vi "AA.vi"(0 "Archivo de\nreferencias (.csv)":path, 5 "ARCHIVO\nTDMS":path, 7 "Largo de ventada temporal en N samples":dbl=44100.0, 9 "Canal":string[](array[string])=["Sound Pressure_0"], 11 "frequency range":T3={"low band"=enum."20 Hz", "high band"=enum."20000 Hz"}) -> (6 "TO CSV.":string[][](array[string]))   [LabVIEW 2017]
uses:
  <vilib>/Waveform/WDTOps.llb/WDT Get Waveform Subset DBL.vi
  <vilib>/addons/Sound and Vibration/svt_Weighting/SVT A, B, C Weighting Filter (Fixed Rates) (1 Ch).vi
  <vilib>/addons/Sound and Vibration/svt_Octave_2014 standard/SVT Third-octave Analysis (1 Ch).vi
  <vilib>/addons/Sound and Vibration/svt_Octave_2014 standard/SVT Weighting Filter (octave) (1 Ch).vi
  <vilib>/addons/Sound and Vibration/svt_Level/SVT Sound Level (1 Ch).vi
  <vilib>/addons/Sound and Vibration/svt_Octave/SoundVib_Octave_2014 standard.lvlib
  <vilib>/addons/Sound and Vibration/svt_Level/SoundVib_SoundLevel.lvlib
  <vilib>/addons/Sound and Vibration/svt_Weighting/SoundVib_ABCWeighting.lvlib
panel:
  in  "reset filter (F)":bool=TRUE
  in  "dB On (T)":bool=TRUE
  in  "restart averaging\n L_bands":bool=TRUE
  in  "exp avg settings":T1={" mode"=enum."Slow", "time constant [ms]"=125.0} {"time constant [ms]" format="%.2f"}
  out "size\nSalida":i32[](array[numeric])
  out "# obs\nBands":i32[](array[numeric])
  out "# obs\nLevels A":i32
  out "total band\npower from 1/3":dbl format="%.2f"
  out "Multiplot \noctave graph 2":T2(graph)
  out "Levels_from SLM":dbl[](array[numeric])
  out "Para el CSV, excepto fecha y hora":string[][](array[string])
  out "ETIQUETAS":string[](array[string])
  out "BANDAS":dbl[][](array[numeric])
  out "Samples \npor Objeto":waveform(dbl)
  out "Secciones":waveform(dbl)[](array[waveform])
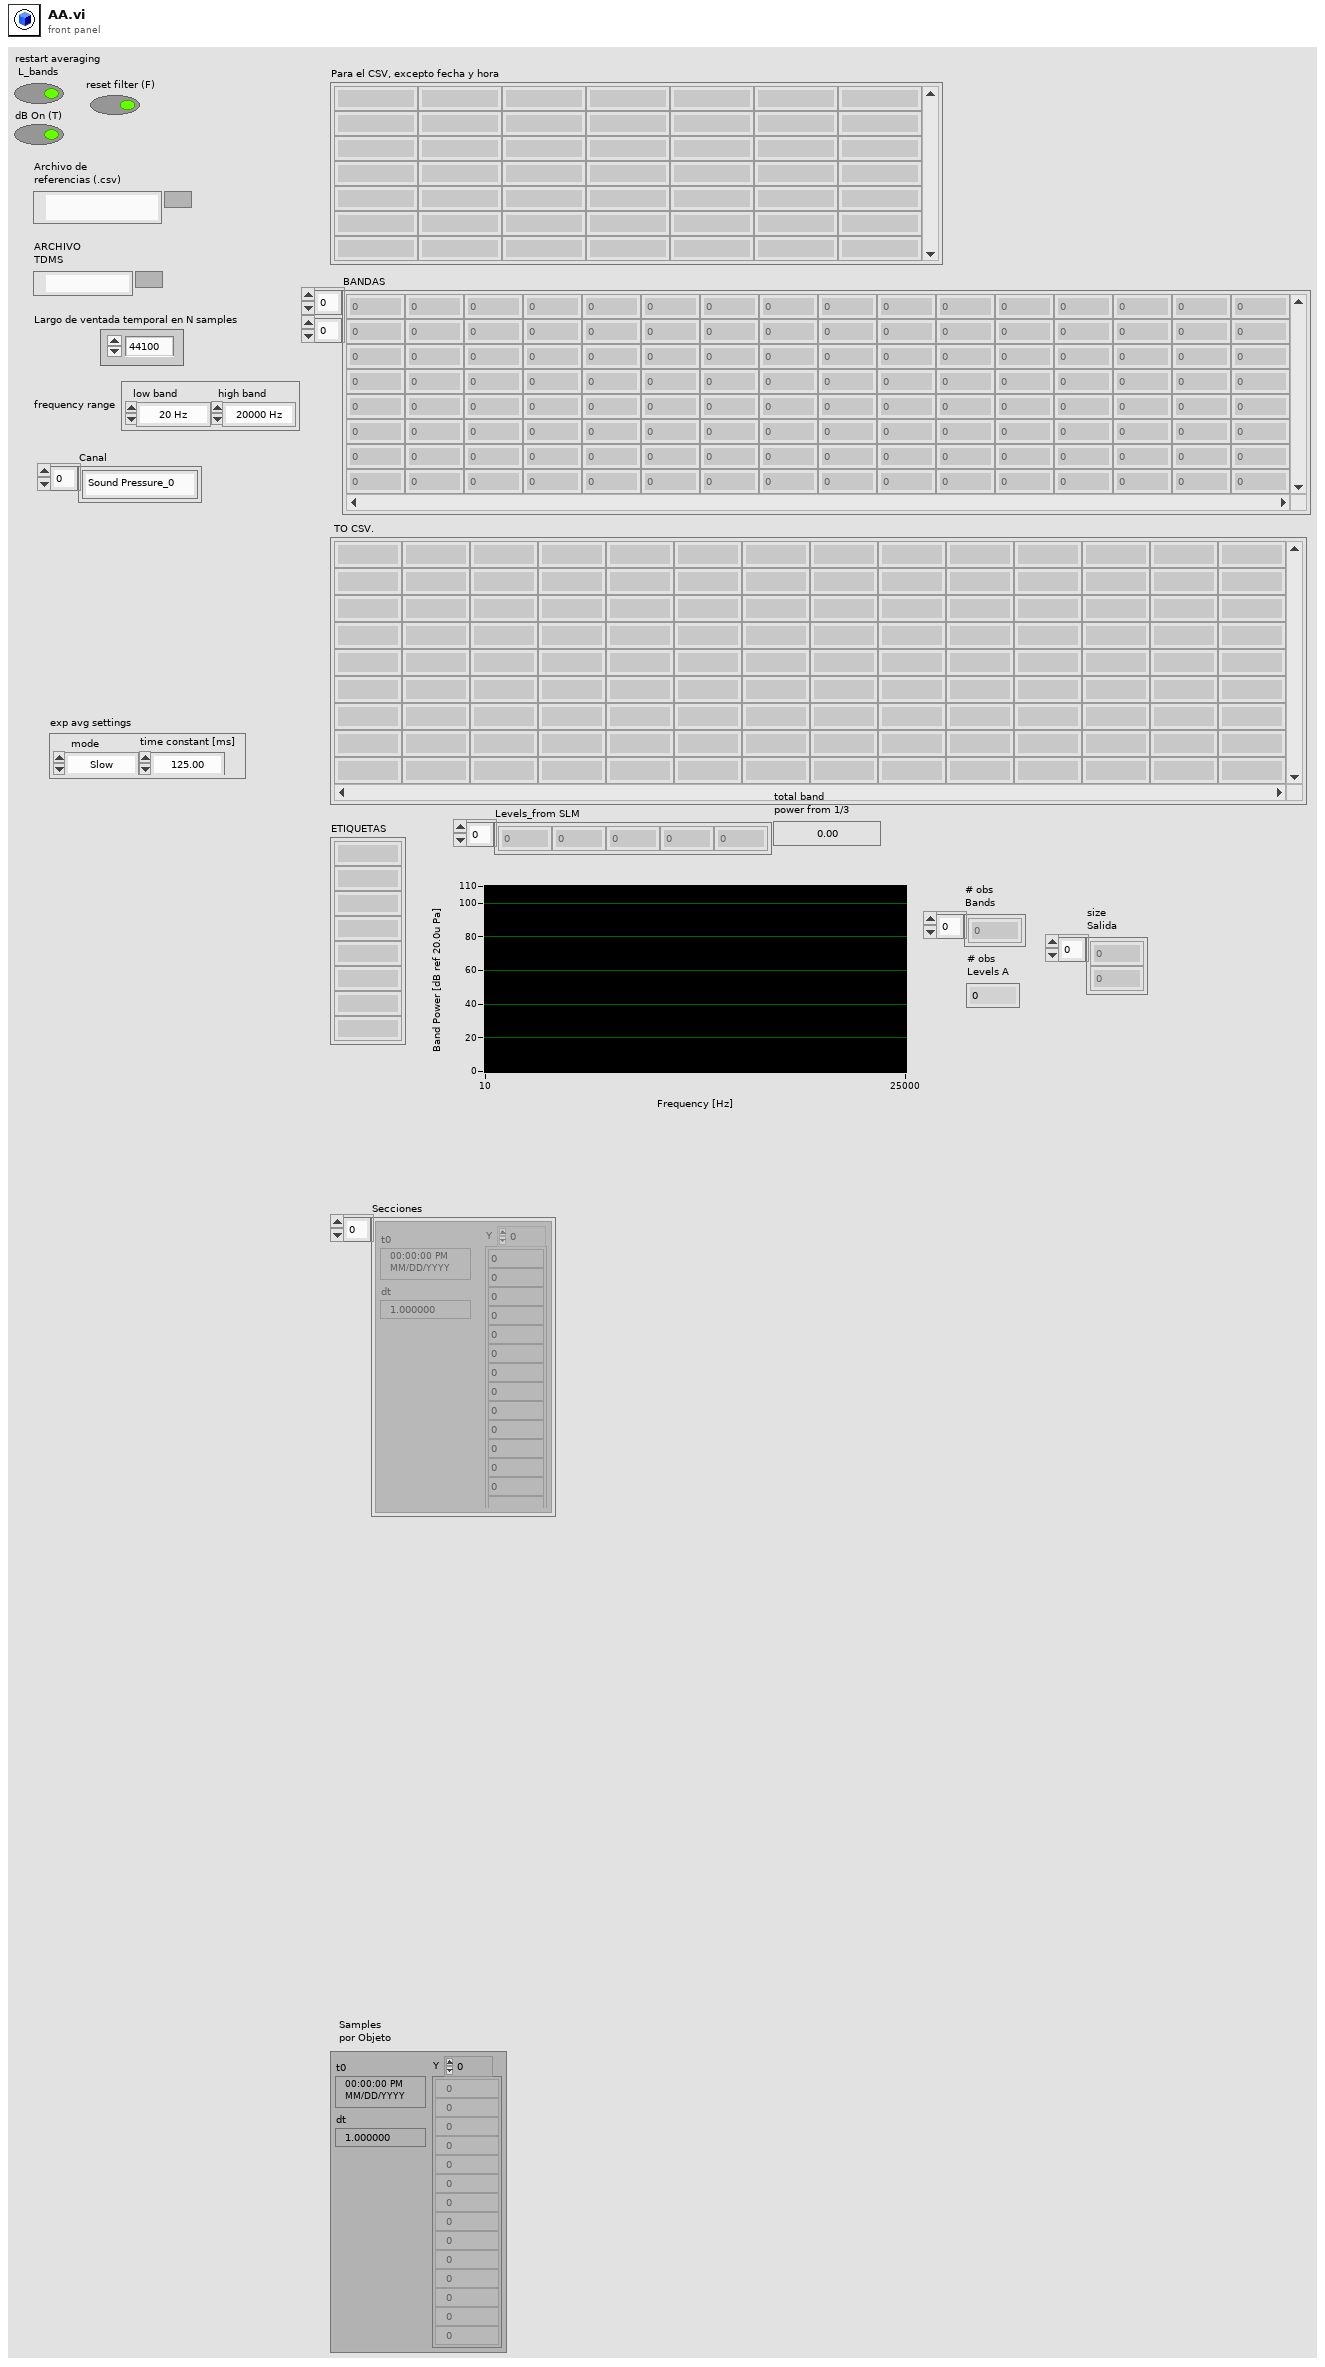
[diagram p1: front panel]
types:
  T1 = cluster{" mode":enum16{"Slow", "Fast", "Impulse", "Custom"}, "time constant [ms]":dbl}
  T2 = cluster{"nominal frequencies [Hz]":dbl[], "band power":dbl[]}
  T3 = cluster{"low band":enum16{"20 Hz", "25 Hz", "31.5 Hz", "40 Hz", "50 Hz", "63 Hz", "80 Hz", "100 Hz", "125 Hz", "160 Hz", "200 Hz", "250 Hz", "315 Hz", "400 Hz", "500 Hz", "630 Hz", "800 Hz", "1000 Hz", "1250 Hz", "1600 Hz", "2000 Hz", "2500 Hz", "3150 Hz", "4000 Hz", "5000 Hz", "6300 Hz", "8000 Hz", "10000 Hz", "12500 Hz", "16000 Hz", "20000 Hz"}, "high band":enum16{"20 Hz", "25 Hz", "31.5 Hz", "40 Hz", "50 Hz", "63 Hz", "80 Hz", "100 Hz", "125 Hz", "160 Hz", "200 Hz", "250 Hz", "315 Hz", "400 Hz", "500 Hz", "630 Hz", "800 Hz", "1000 Hz", "1250 Hz", "1600 Hz", "2000 Hz", "2500 Hz", "3150 Hz", "4000 Hz", "5000 Hz", "6300 Hz", "8000 Hz", "10000 Hz", "12500 Hz", "16000 Hz", "20000 Hz"}}
  T4 = enum16{"open", "open or create", "create or replace", "create", "open (read-only)"}
  T5 = enum16{"Linear", "Exponential", "Equal confidence", "Peak"}
  T6 = cluster{"Leq":bool, "Running Leq":bool, "Exponential":bool, "Peak":bool}
  T7 = typedef "svc_Octave Info.ctl" = cluster{"standard":T8, "bandwidth":enum16{"1 octave", "1/3 octave", "1/6 octave", "1/12 octave", "1/24 octave"}, "low band":i32, "high band":i32, "weighting filter":T9, "dB reference":dbl, "dB On":bool, "unit label":string, "channel name":string, "description":string, "engineering units":T10, "custom label":string, "spectrum type":enum16{"power", "magnitude"}, "spectral density":bool, "filters settled":bool}
  T8 = typedef "svc_Octave Standard.ctl" = enum16{"ANSI S1.11", "IEC 61260"}
  T9 = typedef "svc_Weighting Filter Text Ring.ctl" = u16
  T10 = typedef "svc_Engineering Units Text Ring.ctl" = u16
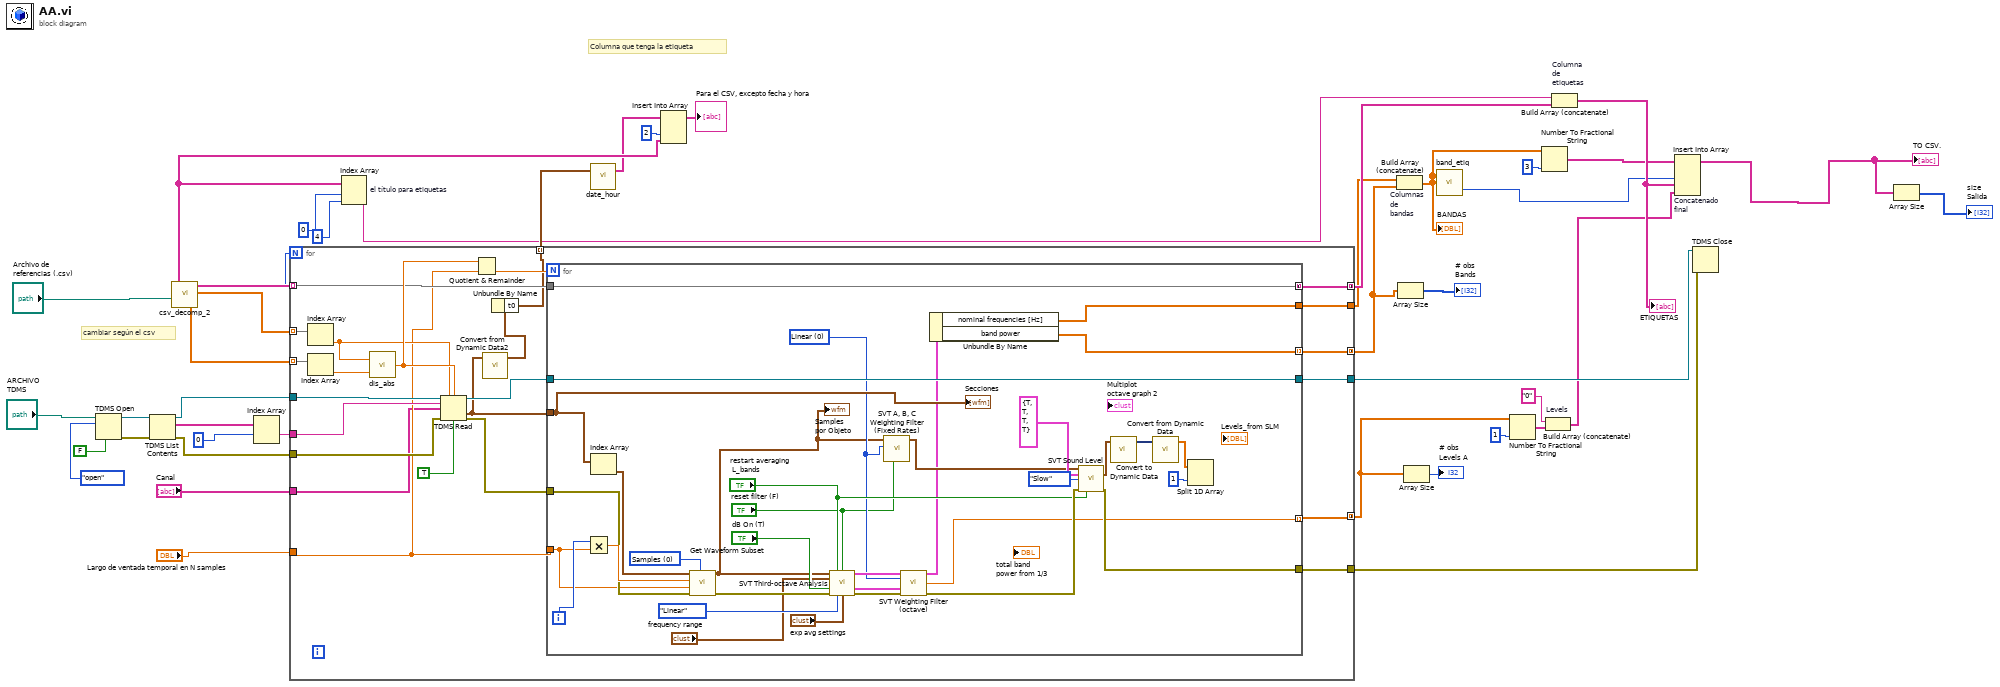
[diagram p0: block diagram]
diagram:
  # "cambiar según el csv"
  # "Columna que tenga la etiqueta"
  n1 = TDMS Open(6:FALSE ("disable buffering? (T)"), 10:T4."open" ("operation (0:open)"), 11:"ARCHIVO\nTDMS") -> (0:w16:errorcluster, 3:w35:refnum<k34>)  [unwired: 4 in]
  n2 = TDMS List Contents(4:w16, 7:w35) -> (0:w37:errorcluster, 2:w36:string[], 3:w17:refnum<k34>)  [unwired: 1 in, 1 out]
  n3 = call "csv_decomp_2.vi"("Archivo de referencias (.csv)"="Archivo de\nreferencias (.csv)") -> ("finales"=w41:dbl[][], "iniciales"=w42:dbl[][], "etiquetas"=w40:string[][], "# dimención"=w11:i32, "Lectura CSV"=w38:string[][])  [unwired: 2 in]
  n4 = Index Array(array=w36, index #1=0 ("index")) -> (element #1=w19:string)  [unwired: 1 in, 1 out]
  n5 = for {
    N: w11 -> [_]
    tunnel: w42 -> [w65] mode=indexing
    tunnel: w41 -> [w66] mode=indexing
    tunnel: w40 -> [w54] mode=indexing
    tunnel: w17 -> [w67]
    tunnel: w37 -> [w60]
    tunnel: w19 -> [w68]
    tunnel: [w58] -> w20
    tunnel: [w57] -> w21
    tunnel: [w56] -> w8 mode=concatenating
    tunnel: [w55] -> w10
    tunnel: [w53] -> w22 mode=concatenating
    tunnel: "Largo de ventada temporal en N samples" -> [w50]
    tunnel: [w47] -> w31 mode=indexing
    tunnel: [w46] -> w6 mode=concatenating
    tunnel: "Canal" -> [w45]
    n6 = Index Array(array=w65) -> (element=w52:dbl)  [unwired: 1 in]
    n7 = Index Array(array=w66) -> (element=w51:dbl)  [unwired: 1 in]
    n8 = call "dis_abs.vi"("Numeric in"=w51, "Numeric 3"=w52) -> ("distancia abs entre dos números"=w61:dbl)
    n9 = TDMS Read(0:w67, 1:w52, 2:w61, 5:w68, 7:w45, 11:w60, 13:TRUE ("return channels in file order? (F)")) -> (4:w64:refnum<k34>, 10:w49:waveform(dbl)[], 15:w59:errorcluster)  [unwired: 1 in, 3 out]
    n10 = Quotient & Remainder(x=w61, y=w50) -> (floor(x/y)=w62:dbl)  [unwired: 1 out]
    n11 = call "Convert from Dynamic Data2"("Dynamic Data Type"=w49) -> ("Waveform"=w48:waveform(dbl))  [unwired: 3 in]
    n12 = Unbundle By Name(w48) -> ("t0"=w47:timestamp)
    n13 = for {
      N: w62 -> [_]
      tunnel: w64 -> [w98]
      tunnel: w49 -> [w92]
      tunnel: w59 -> [w99]
      tunnel: [w91] -> w55
      tunnel: [w98] -> w58
      tunnel: [w97] -> w57
      tunnel: [w96] -> w56 mode=indexing
      tunnel: w54 -> [w95]
      tunnel: [w95] -> w53 mode=concatenating
      tunnel: w50 -> [w93]
      tunnel: [w79] -> w46 mode=indexing
      i -> [w94]
      w73 = u16 0 items=["Linear", "A-weighting", "B-weighting", "C-weighting"] ("weighting")
      w101 = u16 0 items=["Samples", "Relative Time"] ("start/duration format")
      n14 = Multiply(x=w94, y=w93) -> (x*y=w100:dbl)
      n15 = Index Array(array=w92) -> (element=w102:waveform(dbl))  [unwired: 1 in]
      n16 = call-poly <vilib>:"Get Waveform Subset.vi"("start/duration format"=w101, "error in (no error)"=w99, "duration"=w93, "start samples/time"=w100, "waveform in"=w102) -> ("error out"=w86:errorcluster, "waveform out"=w71:waveform(dbl))  [unwired: 1 in, 2 out]
      "Samples \npor Objeto" <- w71
      n17 = call-poly <vilib>:"SVT Third-octave Analysis.vi"("scaled signal [EU]"=w71, "restart averaging (F)"="restart averaging\n L_bands", "reset filter (F)"="reset filter (F)", "frequency range"="frequency range", "dB On (T)"="dB On (T)", "error in (no error)"=w86, "averaging type"=T5."Linear", "exp avg settings"="exp avg settings") -> ("octave spectrum"=w85:T2, "octave info"=w82:T7, "error out"=w84:errorcluster)  [unwired: 2 in, 3 out]
      n18 = call-poly <vilib>:"SVT A, B, C Weighting Filter (Fixed Rates).vi"("reset filter (F)"="reset filter (F)", "weighting"=w73, "scaled signal [EU]"=w71) -> ("weighted signal [EU]"=w70:waveform(dbl))  [unwired: 6 in, 1 out]
      n19 = call-poly <vilib>:"SVT Weighting Filter (octave).vi"("octave spectrum"=w85, "weighting"=w73, "octave info in"=w82, "error in (no error)"=w84) -> ("weighted octave spectrum"=w69:T2, "total band power"=w79:dbl, "error out"=w83:errorcluster)  [unwired: 7 in, 2 out]
      n20 = Unbundle By Name(w69) -> ("nominal frequencies [Hz]"=w97:dbl[], "band power"=w96:dbl[])
      n21 = call-poly <vilib>:"SVT Sound Level.vi"("scaled signal [EU]"=w70, "measurement selection"=T6 {"Leq"=TRUE, "Running Leq"=TRUE, "Exponential"=TRUE, "Peak"=TRUE}, "exponential mode"=enum16{"Slow", "Fast", "Impulse", "Custom"}."Slow", "error in (no error)"=w83, "restart averaging (F)"="restart averaging\n L_bands") -> ("running Leq sound level [dB EU]"=w80:waveform(dbl), "error out"=w91:errorcluster)  [unwired: 5 in, 4 out]
      n22 = call "Convert to Dynamic Data"("Array"=w80) -> ("Dynamic Data Type"=w87:dynamicdata)  [unwired: 3 in]
      n23 = call "Convert from Dynamic Data"("Dynamic Data Type"=w87) -> ("Array"=w89:dbl[])  [unwired: 3 in]
      n24 = Split 1D Array(array=w89, index=1) -> ()  [unwired: 2 out]
      "Secciones" <- w92
    }
  }
  n25 = Index Array "el título para etiquetas"(array=w38, index (row)=0 ("disabled index (row)"), index (col)=4 ("disabled index (col)")) -> (element=w25:string)
  n26 = call "date_hour.vi"("Array"=w31) -> ("appended array"=w32:string[][])  [unwired: 1 in, 1 out]
  n27 = Insert Into Array(array=w32, index (col)=2 ("disabled index (col)"), new element=w38) -> (→"Para el CSV, excepto fecha y hora":string[][])  [unwired: 1 in]
  n28 = Build Array (concatenate) "Columnas \nde\nbandas"(w21, w8) -> (w28:dbl[][])
  "BANDAS" <- w28
  n29 = Array Size(array=w8) -> (size(s)=→"# obs\nBands":i32[])
  n30 = Array Size(array=w6) -> (size(s)=→"# obs\nLevels A":i32)
  n31 = call "band_etiq.vi"("Array de entrada"=w28) -> ("Numeric"=w29:i32)  [unwired: 1 in, 1 out]
  n32 = Number To Fractional String(number=w6, precision (6)=i16 1) -> (F-format string=w4:string[])  [unwired: 2 in]
  n33 = Number To Fractional String(number=w28, precision (6)=i16 3) -> (F-format string=w27:string[][])  [unwired: 2 in]
  n34 = Build Array (concatenate) "Levels"("0", w4) -> (w3:string[])
  n35 = Build Array (concatenate) "Columna \nde \netiquetas"(w25, w22) -> (w44:string[])
  "ETIQUETAS" <- w44
  n36 = Insert Into Array "Concatenado \nfinal"(array=w27, index (col)=w29, new element #1=w44, new element #2=w3) -> (w1:string[][])  [unwired: 1 in]
  "TO CSV." <- w1
  n37 = TDMS Close(8:w10, 11:w20) -> ()  [unwired: 2 out]
  n38 = Array Size(array=w1) -> (size(s)=→"size\nSalida":i32[])
